vi "SQL_EDITOR_check_for_error.vi"(8 "SQL_EDITOR_loop_state_in":T1, 11 "error_in":errorcluster) -> (0 "SQL_EDITOR_loop_state_out":T1, 3 "error_out":errorcluster)   [LabVIEW 2019]
uses:
  SQL_EDITOR_sequence_state.ctl
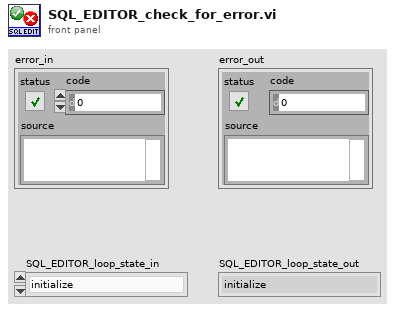
[diagram p1: front panel]
types:
  T1 = typedef "SQL_EDITOR_sequence_state.ctl" = enum16{"initialize", "get_next_state", "REF_read_columns", "REF_read_stations", "REF_select_station_records", "REF_insert_record", "REF_update_record", "REF_delete_record", "REF_send_reference_updated_to_PLC", "ARCH_read_columns", "ARCH_read_stations", "ARCH_select_station_records", "ARCH_insert_record", "ARCH_update_record", "ARCH_delete_record", "USER_read_columns", "USER_select_records", "USER_insert_record", "USER_update_record", "USER_delete_record", "USER_update_barcode", "USER_login", "USER_logout", "SQL_read_tables", "SQL_read_columns", "SQL_select_records", "SQL_insert_record", "SQL_update_record", "SQL_delete_record", "SQL_TEXT_execute", "REPORT_GEAR_scan_barcode", "REPORT_GEAR_get", "REPORT_DATES_get", "REPORT_PBATCH_get", "REPORT_OPRTN_get", "REPORT_CFG_get", "REPORT_AUDIT_get", "REPORT_OKNOK_get", "REPORT_REWORKS_get", "REPORT_PACE_get", "REPORT_CBATCH_scan_barcode", "REPORT_CBATCH_get", "REPORT_CMPNT_scan_barcode", "REPORT_CMPNT_get", "REPORT_save_pdf", "REPORT_save_csv", "error", "stop"}
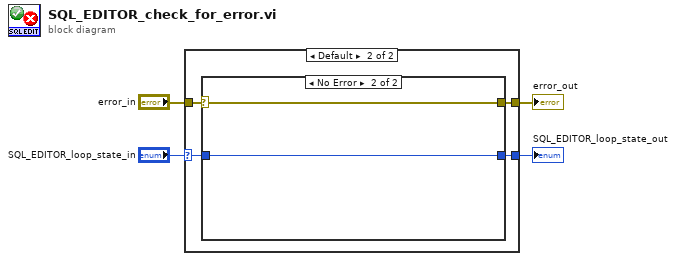
[diagram p0: block diagram]
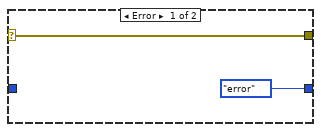
[diagram p3: hidden frame]
diagram:
  n1 = case shown="Default" "SQL_EDITOR_loop_state_in" {
    selector: "SQL_EDITOR_loop_state_in" -> [w5 w8]
    tunnel: [w6 w10] -> w4
    tunnel: [w5 w9] -> w3
    tunnel: "error_in" -> [w6 w7]
    frame "stop" {
    }
    frame Default {
      n2 = case shown="No Error" w7 {
        selector: w7 -> [w12 w13]
        tunnel: [SQL_EDITOR_sequence_state."error" ("PLC_MAIN_loop_state_in") w14] -> w9
        tunnel: w8 -> [_ w14]
        tunnel: [w12 w13] -> w10
        frame Error {
        }
        frame No Error {
        }
      }
    }
  }
  "error_out" <- w4
  "SQL_EDITOR_loop_state_out" <- w3
